vi "Update Move Wait.vi"(8 "error in (no error)":errorcluster, 10 "Tool Buttons":T1, 11 "Map View in":refnum<class "Map View.lvclass">) -> (0 "error out":errorcluster, 3 "Map View out":refnum<class "Map View.lvclass">)   [LabVIEW 2020, in "Map View.lvlib" / "Map View.lvclass"]
uses:
  Map View.lvclass
  Type Definitions/Tool Buttons.ctl
  Map View.lvclass/Map View.ctl
panel:
  # "NOTICE -- YOU MUST LEAVE THIS NOTICE IN PLACE.\n\nCopyright (c) 2017, LIANG LIU Shawn.Liu.cn@gmail.com\nAll rights reserved.\n\nRedistribution and use in source and binary forms, with or without modification, are permitted provided that the following conditions are met:\n-Redistributions of source code must retain the above copyright notice, this list of conditions and the following disclaimer.\n-Redistributions in binary form must reproduce the above copyright notice, this list of conditions and the following disclaimer in the documentation and/or other materials provided with the distribution.\n-Neither the name of the eLp nor the names of its contributors may be used to endorse or promote products derived from this software without specific prior written permission.\n\nTHIS SOFTWARE IS PROVIDED BY THE COPYRIGHT HOLDERS AND CONTRIBUTORS \"AS IS\" AND ANY EXPRESS OR IMPLIED WARRANTIES, INCLUDING, BUT NOT LIMITED TO, THE IMPLIED WARRANTIES OF MERCHANTABILITY AND FITNESS FOR A PARTICULAR PURPOSE ARE DISCLAIMED. IN NO EVENT SHALL THE COPYRIGHT HOLDER OR CONTRIBUTORS BE LIABLE FOR ANY DIRECT, INDIRECT, INCIDENTAL, SPECIAL, EXEMPLARY, OR CONSEQUENTIAL DAMAGES (INCLUDING, BUT NOT LIMITED TO, PROCUREMENT OF SUBSTITUTE GOODS OR SERVICES; LOSS OF USE, DATA, OR PROFITS; OR BUSINESS INTERRUPTION) HOWEVER CAUSED AND ON ANY THEORY OF LIABILITY, WHETHER IN CONTRACT, STRICT LIABILITY, OR TORT (INCLUDING NEGLIGENCE OR OTHERWISE) ARISING IN ANY WAY OUT OF THE USE OF THIS SOFTWARE, EVEN IF ADVISED OF THE POSSIBILITY OF SUCH DAMAGE."
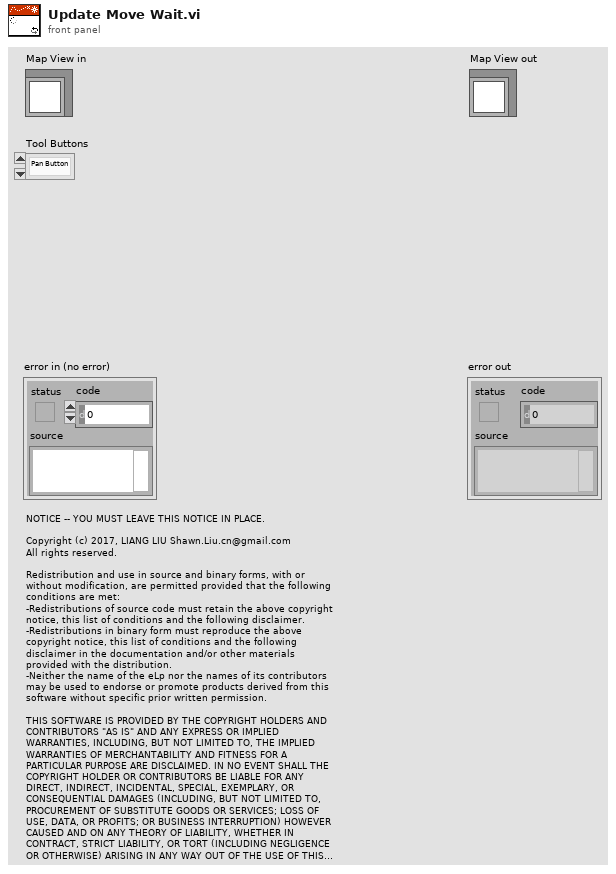
[diagram p1: front panel]
types:
  T1 = typedef "Tool Buttons.ctl" = enum32{"Pan Button", "Pencil Button", "Line Button", "Eraser Button", "Rectangle Select Button", "Deselect Button", "Crop Button", "Rotate Button", "Set Origin Button", "Zoom In Button", "Zoom Out Button"}
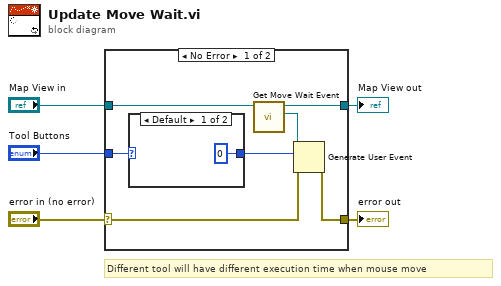
[diagram p0: block diagram]
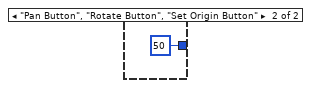
[diagram p2: hidden frame]
diagram:
  # "Different tool will have different execution time when mouse move"
  n1 = case shown="No Error" "error in (no error)" {
    selector: "error in (no error)" -> [w8 w16]
    tunnel: "Map View in" -> [w12 w15]
    tunnel: [w11 w15] -> w4
    tunnel: "Tool Buttons" -> [w10 _]
    tunnel: [w6 w16] -> w1
    frame No Error {
      n2 = case shown="Default" w10 {
        tunnel: [u32 0 u32 50] -> w9
        frame Default {
        }
        frame "Pan Button", "Rotate Button", "Set Origin Button" {
        }
      }
      n3 = call "Get Move Wait Event.vi"("Map View in"=w12) -> ("Move Wait Event"=w7:refnum<user-event>, "Map View out"=w11:refnum<class "Map View.lvclass">)  [unwired: 9 in]
      n4 = Generate User Event(user event=w7, event data cluster=w9, error in=w8) -> (error out=w6:errorcluster)  [unwired: 1 in, 1 out]
    }
    frame Error {
    }
  }
  "error out" <- w1
  "Map View out" <- w4
